vi "TestExec.Test ID - Update Section.vi"(9 "TC Level":i32, 10 "TC Cnts":i32[](array[numeric]), 11 "Start(T)/End(F)":bool) -> (0 "Test ID":string, 1 "TC Level Out":i32, 2 "TC Cnts Out":i32[](array[numeric]))   [LabVIEW 2016]
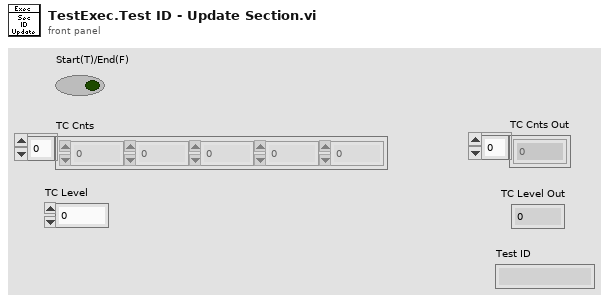
[diagram p1: front panel]
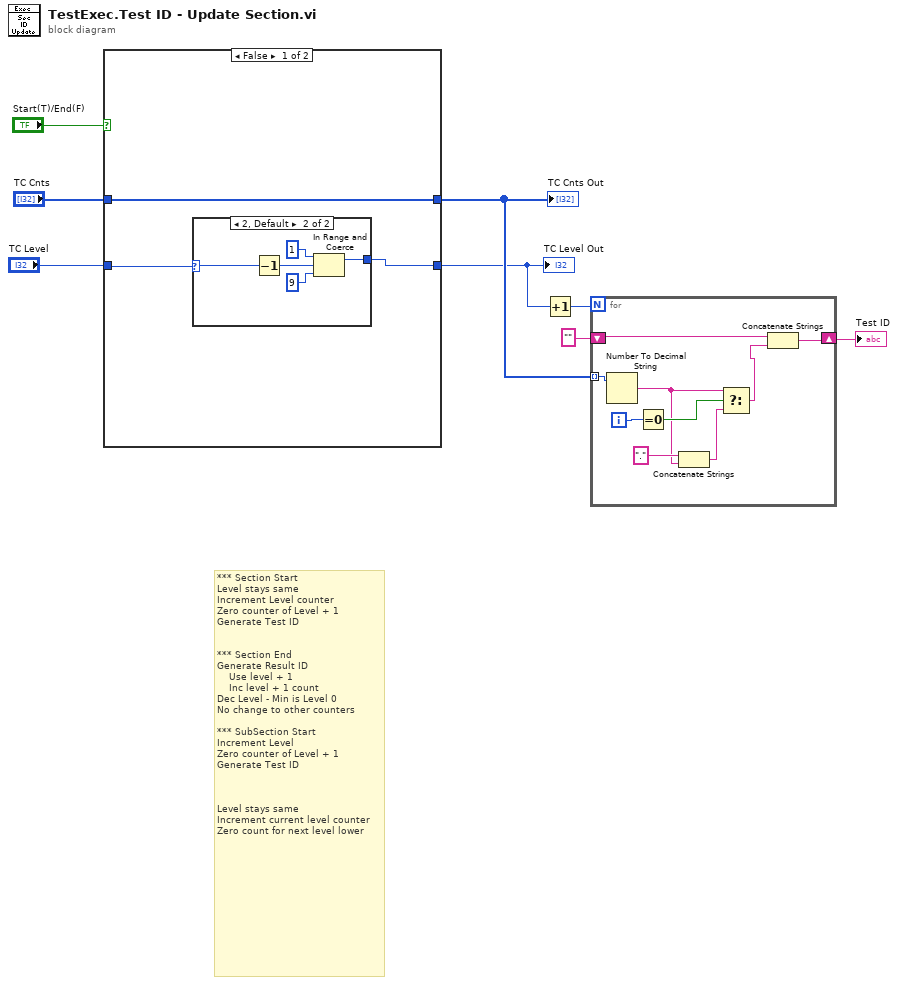
[diagram p0: block diagram]
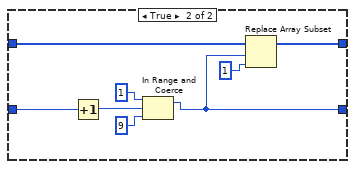
[diagram p3: hidden frame]
diagram:
  # "*** Section Start\nLevel stays same\nIncrement Level counter\nZero counter of Level + 1\nGenerate Test ID\n\n\n*** Section End\nGenerate Result ID\n    Use level + 1\n    Inc level + 1 count\nDec Level - Min is Level 0\nNo change to other counters\n\n*** SubSection Start\nIncrement Level\nZero counter of Level + 1\nGenerate Test ID\n\n\n\nLevel stays same\nIncrement current level counter\nZero count for next level lower"
  n1 = case shown="False" "Start(T)/End(F)" {
    tunnel: "TC Cnts" -> [w11 w24]
    tunnel: "TC Level" -> [w9 w23]
    tunnel: [w11 w22] -> w5
    tunnel: [w10 w18] -> w3
    frame False {
      n2 = case shown="2, Default" w9 {
        selector: w9 -> [w12 w13]
        tunnel: [w12 w14] -> w10
        frame 0, 1 {
          # "Do Nothing"
        }
        frame 2, Default {
          n3 = Decrement(x=w13) -> (x-1=w17:i32)
          n4 = In Range and Coerce(upper limit=1, x=w17, lower limit=9 ("upper limit")) -> (coerced(x)=w14:i32)  [unwired: 1 out]
        }
      }
    }
    frame True {
      n5 = Increment(x=w23) -> (x+1=w19:i32)
      n6 = In Range and Coerce(upper limit=1, x=w19, lower limit=9 ("upper limit")) -> (coerced(x)=w18:i32)  [unwired: 1 out]
      n7 = Replace Array Subset(array=w24, new element=1, index=w18) -> (w22:i32[])
    }
  }
  "TC Cnts Out" <- w5
  "TC Level Out" <- w3
  n8 = Increment(x=w3) -> (x+1=w4:i32)
  n9 = for {
    N: w4 -> [_]
    tunnel: w5 -> [w33] mode=indexing
    shift-right: [w28] -> w1
    shift-left: "" -> [w27]
    i -> [w34]
    n10 = Number To Decimal String(number=w33) -> (decimal integer string=w29:string)  [unwired: 1 in]
    n11 = Equal To 0?(x=w34) -> (x = 0?=w30:bool)
    n12 = Concatenate Strings(".", w29) -> (w31:string)
    n13 = Select(t=w29, s=w30, f=w31) -> (s? t:f=w26:string)
    n14 = Concatenate Strings(w27, w26) -> (w28:string)
  }
  "Test ID" <- w1
